vi "OpenConnection.vi"(0 "STOMP in":refnum<class "STOMP.lvclass">, 1 "address":string="localhost", 2 "port":u16=61613, 4 "timeout ms (60000)":i32, 5 "error in (no error)":errorcluster) -> (14 "STOMP out":refnum<class "STOMP.lvclass">, 19 "error out":errorcluster)   [LabVIEW 2017, in "LabVIEW STOMP.lvlib" / "STOMP.lvclass"]
uses:
  STOMP.lvclass
  STOMP.lvclass/STOMP.ctl
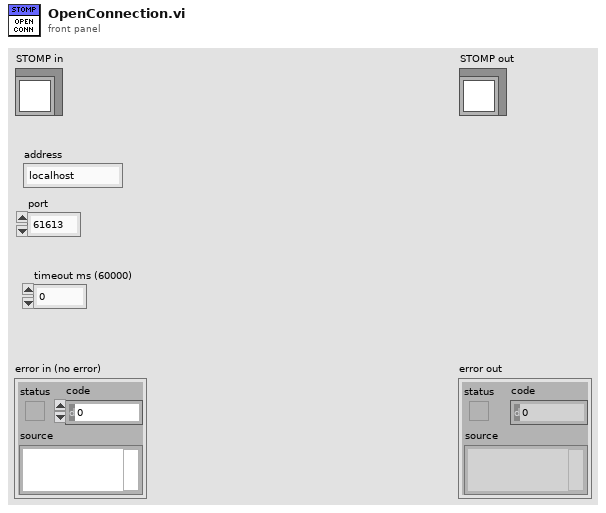
[diagram p1: front panel]
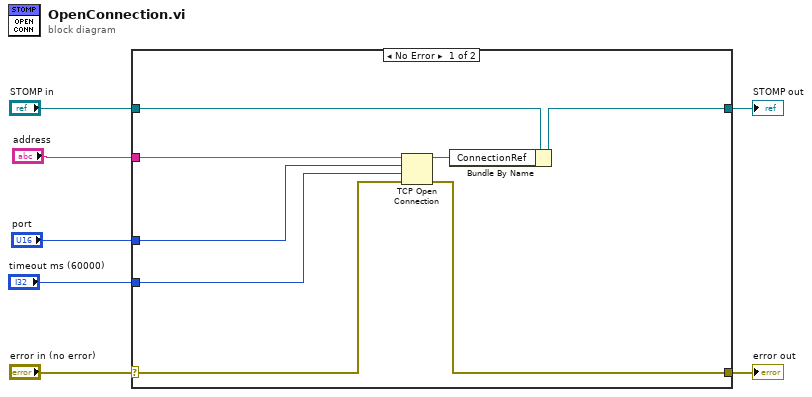
[diagram p0: block diagram]
diagram:
  n1 = case shown="No Error" "error in (no error)" {
    selector: "error in (no error)" -> [w9 w17]
    tunnel: [w8 w17] -> w6
    tunnel: [w10 w16] -> w4
    tunnel: "STOMP in" -> [w11 w16]
    tunnel: "timeout ms (60000)" -> [w14 _]
    tunnel: "port" -> [w13 _]
    tunnel: "address" -> [w12 _]
    frame No Error {
      n2 = TCP Open Connection(address=w12, remote port or service name=w13, timeout ms (60000)=w14, error in (no error)=w9) -> (connection ID=w15:refnum<k5>, error out=w8:errorcluster)  [unwired: 1 in]
      n3 = Bundle By Name(cluster=w11, "ConnectionRef"=w15) -> (w10:refnum<class "STOMP.lvclass">)
    }
    frame Error {
    }
  }
  "error out" <- w6
  "STOMP out" <- w4
